vi "PickedObjects.vi"(8 "error in (no error)":errorcluster, 10 "Point":T1, 11 "Control Window in":refnum<class "Control Window.lvclass">) -> (0 "error out":errorcluster, 2 "Objects":refnum<class "3D Object.lvclass">[](array[class]), 3 "Control Window out":refnum<class "Control Window.lvclass">)   [LabVIEW 2015, in "Control Window.lvclass"]
uses:
  Control Window.lvclass
  <vilib>/Utility/miscctls.llb/LVPoint32TypeDef.ctl
  3D Object/3D Object.lvclass
  Control Window.lvclass/Control Window.ctl
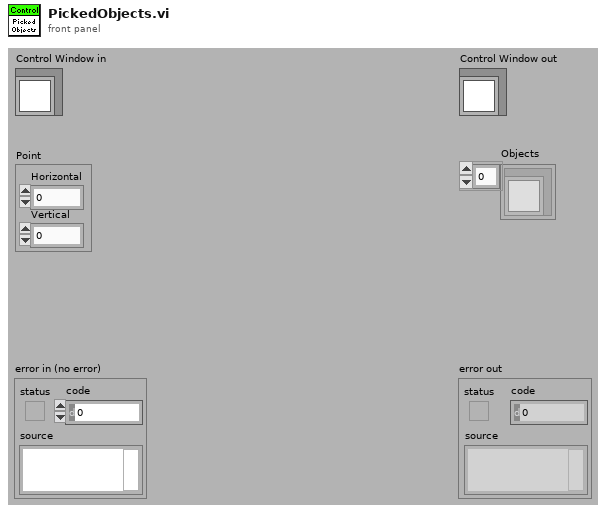
[diagram p1: front panel]
types:
  T1 = typedef "LVPoint32TypeDef.ctl" = cluster{"Horizontal":i32, "Vertical":i32}
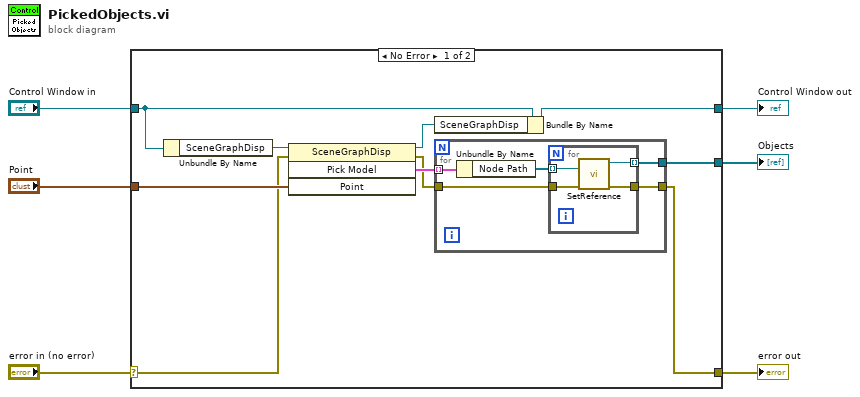
[diagram p0: block diagram]
diagram:
  n1 = case shown="No Error" "error in (no error)" {
    selector: "error in (no error)" -> [w9 w27]
    tunnel: [w8 w27] -> w5
    tunnel: [w16 w26] -> w3
    tunnel: "Control Window in" -> [w12 w26]
    tunnel: "Point" -> [w10 _]
    tunnel: [w7 _] -> w1
    frame No Error {
      n2 = Unbundle By Name(w12) -> ("SceneGraphDisp"=w11:refnum<vi>)
      n3 = invoke class="SceneGraphDisp" method="Pick Model"(reference=w11, error in=w9, "Point"=w10) -> (reference out=w15:refnum<vi>, error out=w13:errorcluster, "Pick Model"=w14:cluster{"Node Path":refnum<vi>[]}[])  [unwired: 1 in, 1 out]
      n4 = Bundle By Name(cluster=w12, "SceneGraphDisp"=w15) -> (w16:refnum<class "Control Window.lvclass">)
      n5 = for {
        tunnel: w14 -> [w21] mode=indexing
        tunnel: w13 -> [w19]
        tunnel: [w18] -> w7
        tunnel: [w17] -> w8
        n6 = Unbundle By Name(w21) -> ("Node Path"=w20:refnum<vi>[])
        n7 = for {
          tunnel: w20 -> [w25] mode=indexing
          tunnel: w19 -> [w24]
          tunnel: [w23] -> w18 mode=indexing
          tunnel: [w22] -> w17
          n8 = call "SetReference.vi"("error in (no error)"=w24, "SceneObject"=w25) -> ("error out"=w22:errorcluster, "3D Object out"=w23:refnum<class "3D Object.lvclass">)  [unwired: 8 out]
        }
      }
    }
    frame Error {
    }
  }
  "error out" <- w5
  "Control Window out" <- w3
  "Objects" <- w1
